vi "Disconnect.vi"(8 "error in (no error)":errorcluster, 11 ".NET Refnum in":refnum<k24>) -> ()   [LabVIEW 2024, in "LV_OPC_NET.lvlib"]
uses:
  C:/Users/Andrey/Desktop/LV_OPC-Client-x64/LV_OPC_Test/OPC.NET/OpcNetApi.dll
  OpcNetApi.dll
  LV_OPC_NET.lvlib
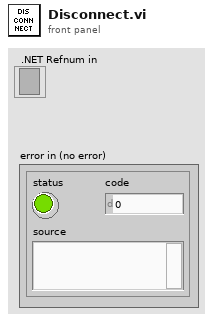
[diagram p1: front panel]
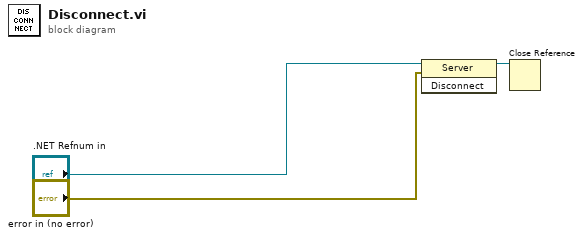
[diagram p0: block diagram]
diagram:
  n1 = invoke class="Server" method="Disconnect"(reference=".NET Refnum in", error in="error in (no error)") -> (reference out=w2:refnum<k24>)  [unwired: 1 in, 2 out]
  n2 = Close Reference(reference=w2) -> ()  [unwired: 1 in, 1 out]
